vi "NI9219_CREATE_TASK.vi"(8 "error in":errorcluster) -> (0 "error out":errorcluster, 3 "task out":refnum<k21>)   [LabVIEW 2022 SP3]
uses:
  <vilib>/DAQmx/create/channels.llb/DAQmx Create Channel (AI-Voltage-Basic).vi
  <vilib>/DAQmx/create/channels.llb/DAQmx Create Channel (AI-Current-Basic).vi
  <resource>/objmgr/daqmx.rc
  <vilib>/DAQmx/configure/timing.llb/DAQmx Timing (Sample Clock).vi
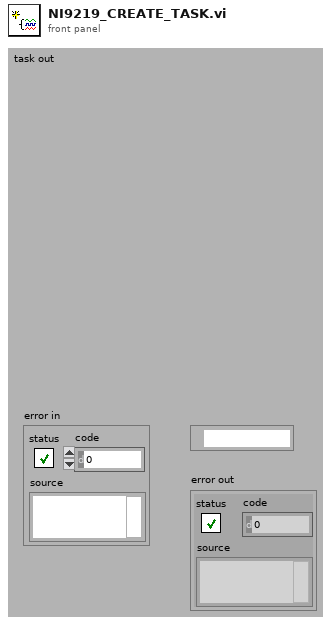
[diagram p1: front panel]
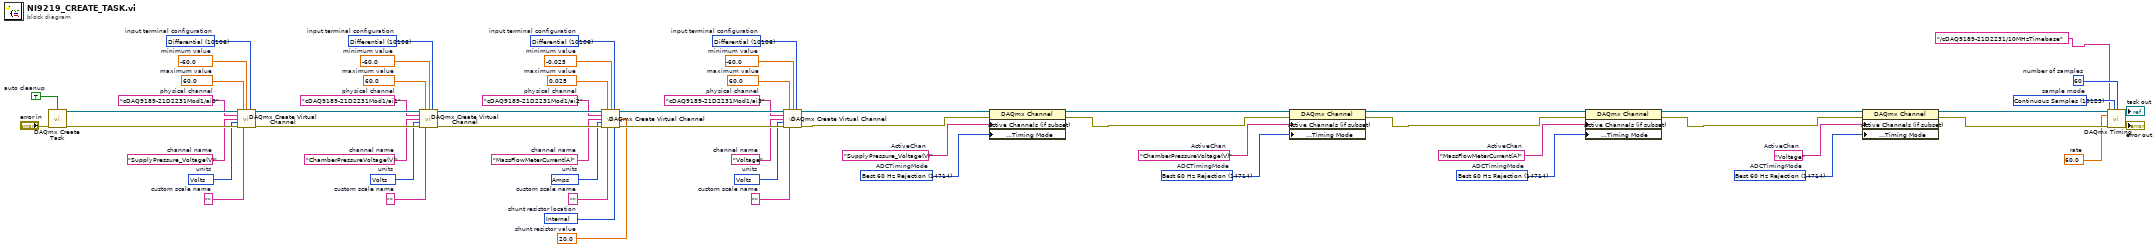
[diagram p0: block diagram]
diagram:
  w2 = 10123 items=["Finite Samples"=10178, "Continuous Samples"=10123, "Hardware Timed Single Point"=12522]  # sample mode
  w3 = 60  # number of samples
  w4 = 60.0  # rate
  w9 = 14714 items=["High Resolution"=10195, "High Speed"=14712, "Best 50 Hz Rejection"=14713, "Best 60 Hz Rejection"=14714]  # ADCTimingMode
  w11 = "Voltage"  # ActiveChan
  w13 = 14714 items=["High Resolution"=10195, "High Speed"=14712, "Best 50 Hz Rejection"=14713, "Best 60 Hz Rejection"=14714]  # ADCTimingMode
  w15 = "MassFlowMeterCurrent(A)"  # ActiveChan
  w17 = 14714 items=["High Resolution"=10195, "High Speed"=14712, "Best 50 Hz Rejection"=14713, "Best 60 Hz Rejection"=14714]  # ADCTimingMode
  w19 = "ChamberPressureVoltage(V)"  # ActiveChan
  w21 = 14714 items=["High Resolution"=10195, "High Speed"=14712, "Best 50 Hz Rejection"=14713, "Best 60 Hz Rejection"=14714]  # ADCTimingMode
  w23 = "SupplyPressure_Voltage(V)"  # ActiveChan
  w24 = 10106 items=["default"=-1, "RSE"=10083, "NRSE"=10078, "Differential"=10106, "Pseudodifferential"=12529]  # input terminal configuration
  w25 = 10348 items=["Volts"=10348, "From Custom Scale"=10065]  # units
  w26 = "Voltage"  # channel name
  w28 = ""  # custom scale name
  w29 = -60.0  # minimum value
  w30 = 60.0  # maximum value
  w31 = "cDAQ9189-21D2231Mod1/ai3"  # physical channel
  w33 = 10106 items=["default"=-1, "RSE"=10083, "NRSE"=10078, "Differential"=10106, "Pseudodifferential"=12529]  # input terminal configuration
  w34 = 10342 items=["Amps"=10342, "From Custom Scale"=10065]  # units
  w35 = 20.0  # shunt resistor value
  w36 = 10200 items=["Internal"=10200, "External"=10167]  # shunt resistor location
  w37 = "MassFlowMeterCurrent(A)"  # channel name
  w39 = ""  # custom scale name
  w40 = -0.025  # minimum value
  w41 = 0.025  # maximum value
  w42 = "cDAQ9189-21D2231Mod1/ai2"  # physical channel
  w44 = 10106 items=["default"=-1, "RSE"=10083, "NRSE"=10078, "Differential"=10106, "Pseudodifferential"=12529]  # input terminal configuration
  w45 = 10348 items=["Volts"=10348, "From Custom Scale"=10065]  # units
  w46 = "ChamberPressureVoltage(V)"  # channel name
  w48 = ""  # custom scale name
  w49 = -60.0  # minimum value
  w50 = 60.0  # maximum value
  w51 = "cDAQ9189-21D2231Mod1/ai1"  # physical channel
  w53 = 10106 items=["default"=-1, "RSE"=10083, "NRSE"=10078, "Differential"=10106, "Pseudodifferential"=12529]  # input terminal configuration
  w54 = 10348 items=["Volts"=10348, "From Custom Scale"=10065]  # units
  w55 = "SupplyPressure_Voltage(V)"  # channel name
  w57 = ""  # custom scale name
  w58 = -60.0  # minimum value
  w59 = 60.0  # maximum value
  w60 = "cDAQ9189-21D2231Mod1/ai0"  # physical channel
  w62 = TRUE  # auto cleanup
  n1 = call <vilib>:"DAQmx Create Task.vi"("auto cleanup"=w62, "error in"="error in") -> ("task out"=w61:refnum<k21>, "error out"=w63:errorcluster)  [unwired: 12 in]
  n2 = call-poly <vilib>:"DAQmx Create Virtual Channel.vi"("task in"=w61, "maximum value"=w59, "minimum value"=w58, "input terminal configuration"=w53, "physical channels"=w60, "name to assign"=w55, "units"=w54, "error in"=w63, "custom scale name"=w57) -> ("task out"=w52:refnum<k21>, "error out"=w56:errorcluster)  [unwired: 5 in]
  n3 = call-poly <vilib>:"DAQmx Create Virtual Channel.vi"("task in"=w52, "maximum value"=w50, "minimum value"=w49, "input terminal configuration"=w44, "physical channels"=w51, "name to assign"=w46, "units"=w45, "error in"=w56, "custom scale name"=w48) -> ("task out"=w43:refnum<k21>, "error out"=w47:errorcluster)  [unwired: 5 in]
  n4 = call-poly <vilib>:"DAQmx Create Virtual Channel.vi"("task in"=w43, "maximum value"=w41, "minimum value"=w40, "input terminal configuration"=w33, "physical channels"=w42, "name to assign"=w37, "external shunt resistor value"=w35, "units"=w34, "error in"=w47, "custom scale name"=w39, "shunt resistor location"=w36) -> ("task out"=w32:refnum<k21>, "error out"=w38:errorcluster)  [unwired: 3 in]
  n5 = call-poly <vilib>:"DAQmx Create Virtual Channel.vi"("task in"=w32, "maximum value"=w30, "minimum value"=w29, "input terminal configuration"=w24, "physical channels"=w31, "name to assign"=w26, "units"=w25, "error in"=w38, "custom scale name"=w28) -> ("task out"=w20:refnum<k21>, "error out"=w27:errorcluster)  [unwired: 5 in]
  n6 = property class="DAQmx Channel"(reference=w20, error in=w27, "Active Channels (if subset)"=w23, "Analog Input:General Properties:Digitizer/ADC:Timing Mode"=w21) -> (reference out=w16:refnum<k21>, error out=w22:errorcluster)
  n7 = property class="DAQmx Channel"(reference=w16, error in=w22, "Active Channels (if subset)"=w19, "Analog Input:General Properties:Digitizer/ADC:Timing Mode"=w17) -> (reference out=w12:refnum<k21>, error out=w18:errorcluster)
  n8 = property class="DAQmx Channel"(reference=w12, error in=w18, "Active Channels (if subset)"=w15, "Analog Input:General Properties:Digitizer/ADC:Timing Mode"=w13) -> (reference out=w8:refnum<k21>, error out=w14:errorcluster)
  n9 = property class="DAQmx Channel"(reference=w8, error in=w14, "Active Channels (if subset)"=w11, "Analog Input:General Properties:Digitizer/ADC:Timing Mode"=w9) -> (reference out=w5:refnum<k21>, error out=w10:errorcluster)
  n10 = call-poly <vilib>:"DAQmx Timing.vi"("task/channels in"=w5, "sample mode"=w2, "samples per channel"=w3, "rate"=w4, "source"=tag "/cDAQ9189-21D2231/10MHzTimebase", "error in"=w10) -> ("task out"=→"task out":refnum<k21>, "error out"=→"error out":errorcluster)  [unwired: 8 in]
